vi "Actor Core.vi"(8 "error in":errorcluster, 11 "Stage":refnum<class "Stage.lvclass">) -> (0 "error out":errorcluster, 3 "Actor out":refnum<class "Actor.lvclass">)   [LabVIEW 2018, in "Stage Actor.lvlib" / "Stage.lvclass"]
doc: "This is Actor Core.vi, the main message handling loop for Actors. An actor usually just sits in this loop and processes messages as they arrive. Any error returned by the message Do.vi call will stop the loop, with error code 43 as the canonical signal to stop with no error sent to caller. Descendants may override that in Handle Error.vi."
uses:
  Stage.lvclass
  C:/Program Files (x86)/National Instruments/LabVIEW 2018/vi.lib/MGI/Panel Manager/Panel Actor/Panel Actor/Panel Actor.lvclass
  C:/Program Files (x86)/National Instruments/LabVIEW 2018/vi.lib/ActorFramework/Actor/Actor.lvclass
  <vilib>/ActorFramework/Actor/Actor.lvclass
  Stage.lvclass/Stage.ctl
  <vilib>/ActorFramework/Actor/Actor.lvclass/Actor.ctl
  <vilib>/ActorFramework/Message Enqueuer/Message Enqueuer.lvclass/Message Enqueuer.ctl
  Stage Messages/Set Axis Speed Msg/Set Axis Speed Msg.lvclass/Set Axis Speed Msg.ctl
  Stage Messages/Move to Position Msg/Move to Position Msg.lvclass/Move to Position Msg.ctl
  Stage Messages/Parse Gcode Msg/Parse Coords Msg.lvclass/Parse Coords Msg.ctl
  <vilib>/ActorFramework/Message Enqueuer/Init from Existing Queue.vi
  <vilib>/ActorFramework/Message Enqueuer/Enqueue.vi
  Stage Messages/Stop Stage Msg/Stop Stage Msg.lvclass
  C:/Program Files (x86)/National Instruments/LabVIEW 2018/vi.lib/ActorFramework/Message/Message.lvclass
  Stage Messages/Set Axis Speed Msg/Set Axis Speed Msg.lvclass
  Stage Messages/Home Stage Msg/Home Stage Msg.lvclass
  Stage Messages/Move to Position Msg/Move to Position Msg.lvclass
  Stage Messages/Test VI Msg/Test VI Msg.lvclass
  Stage Messages/Parse Gcode Msg/Parse Coords Msg.lvclass
  <vilib>/ActorFramework/Message Priority Queue/Priority Enqueue.vi
  <vilib>/ActorFramework/Message Enqueuer/Message Enqueuer.lvclass
  <vilib>/MGI/Panel Manager/Panel Actor/Panel Actor/Panel Actor.lvclass
  ADM/Main.lvlib
  <instrlib>/Zaber A Series/Zaber A Series.lvlib
  Stage Messages/Stage Polling Loop Msg/Stage Polling Loop Msg.lvclass
  Stage Messages/Stage Printing Loop Msg/Stage Printing Loop Msg.lvclass
panel:
  in  "Apply Movement":bool
  in  "Travel to Saved":bool
  in  "Save Position":bool
  in  "Move to Specified Position":dbl[](array[numeric])
  out "Saved Position":dbl[](array[numeric])
  in  "Z Speed(mm/s)":dbl(slide)=0.09999999999999998 min=0.0 max=10.0 step=0.01 scale=0.01..10.0
  in  "XY Speed":i16(ring)=10 items=["Fast"=10, "Slow"=1]
  in  "Cancel Button":bool
  in  "Print":bool
  in  "Read Coordinates":path
  in  "-Z":bool
  in  "+Z":bool
  in  "Home Button":bool
  in  "-X":bool
  in  "+X":bool
  in  "-Y":bool
  in  "+Y":bool
  out "Current Position":dbl[](array[numeric])
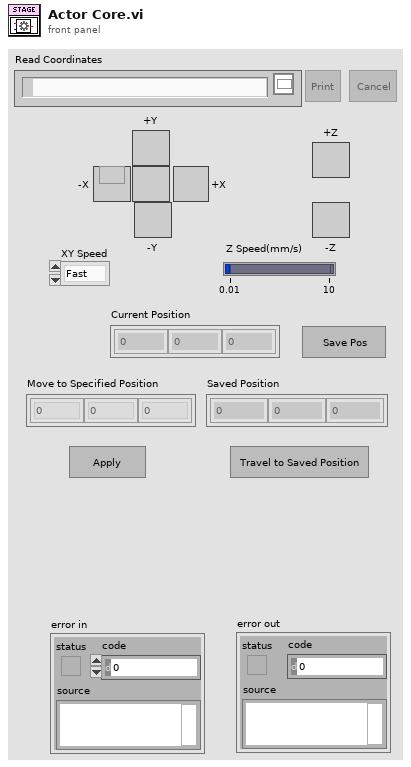
[diagram p1: front panel]
types:
  T1 = cluster{"Print Data":cluster{"XYZ":dbl[][], "Theta Phi":dbl[][], "Current Tool":i16[], "Speed":dbl[], "Feeder State":bool[]}, "Task":string}
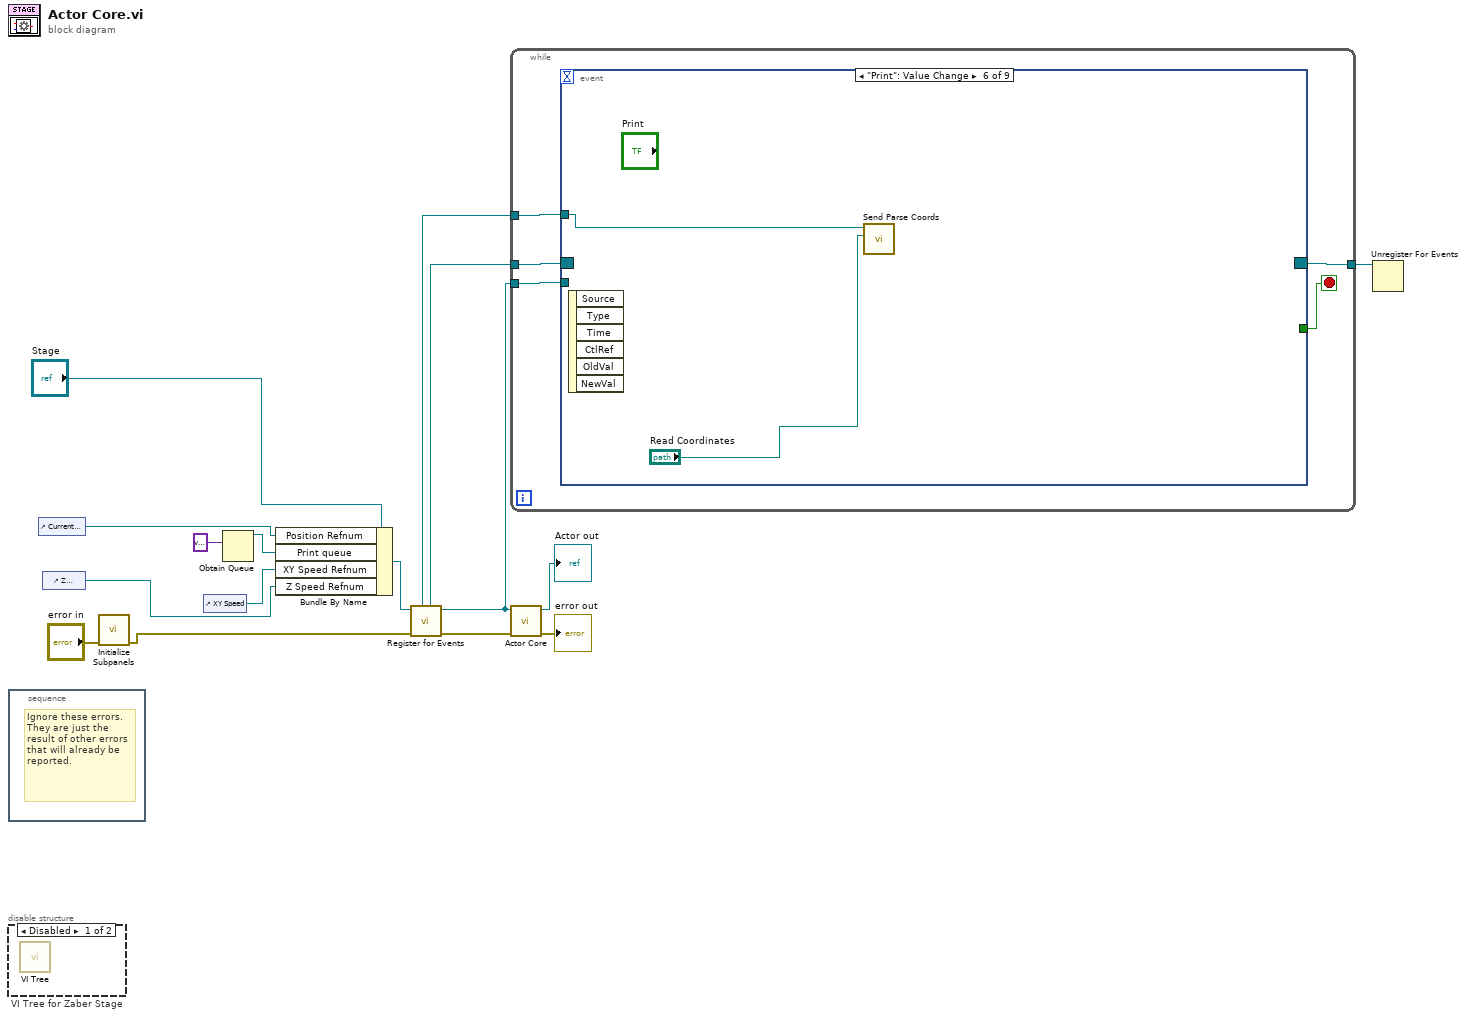
[diagram p0: block diagram]
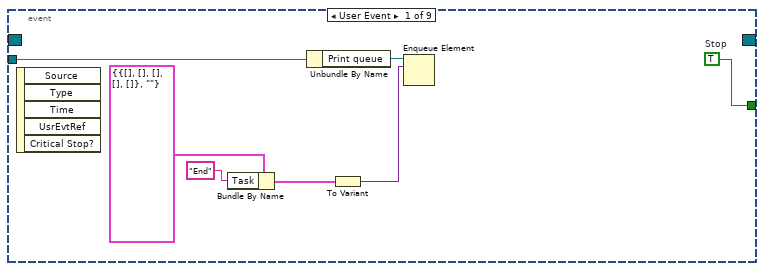
[diagram p2: hidden frame]
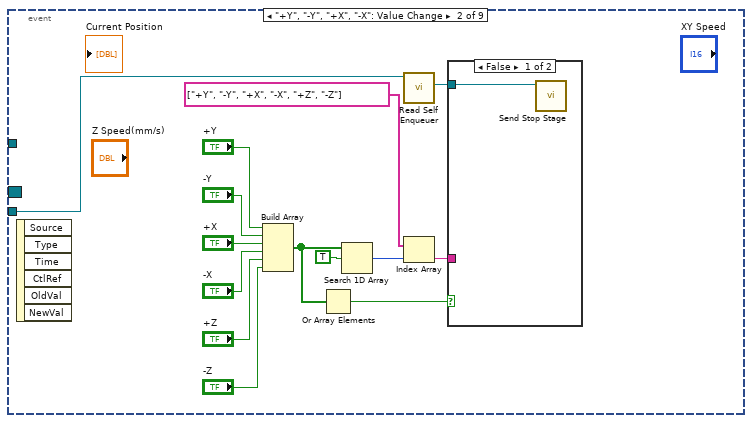
[diagram p3: hidden frame]
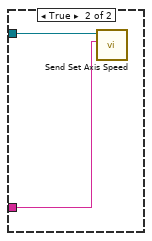
[diagram p4: hidden frame]
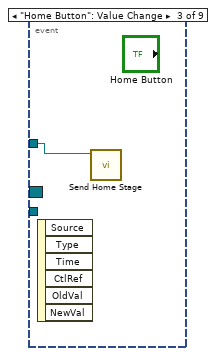
[diagram p5: hidden frame]
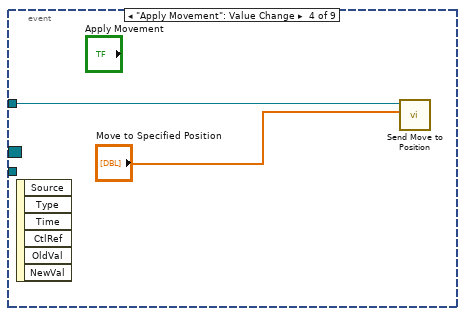
[diagram p6: hidden frame]
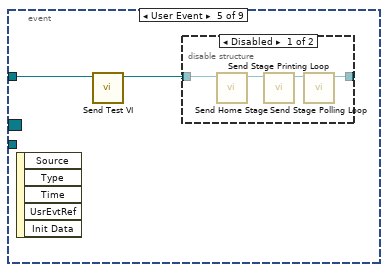
[diagram p7: hidden frame]
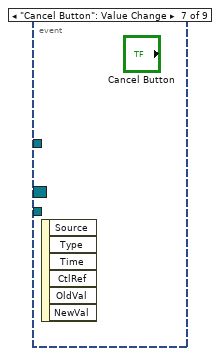
[diagram p9: hidden frame]
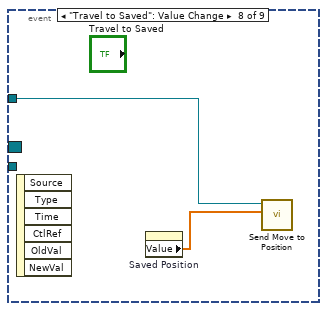
[diagram p10: hidden frame]
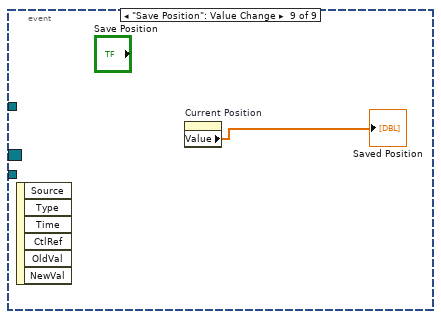
[diagram p11: hidden frame]
diagram:
  n1 = stacked-sequence {
    frame #0 {
      # "Ignore these errors.\nThey are just the result of other errors that will already be reported."
    }
  }
  n2 = disable-structure "VI Tree for Zaber Stage" shown="Disabled" {
    frame Disabled {
      n3 = call <instrlib>:"VI Tree.vi"() -> ()  [unwired: 12 in]
    }
    frame Enabled {
    }
  }
  n4 = control-ref of="Current Position"() -> (w12:refnum<vi>)
  n5 = control-ref of="Z Speed(mm/s)"() -> (w8:refnum<vi>)
  n6 = call "Initialize Subpanels.vi"("error in (no error)"="error in") -> ("error out"=w1:errorcluster)  [unwired: 10 in]
  n7 = control-ref of="XY Speed"() -> (w9:refnum<vi>)
  n8 = Obtain Queue(element data type=variant) -> (queue out=w11:refnum<queue>)  [unwired: 4 in, 2 out]
  n9 = Bundle By Name(cluster="Stage", "Position Refnum"=w12, "Print queue"=w11, "XY Speed Refnum"=w9, "Z Speed Refnum"=w8) -> (w6:refnum<class "Stage.lvclass">)
  n10 = call <vilib>:"Register for Events.vi"("Error In"=w1, "Panel Actor in"=w6) -> ("Error Out"=w5:errorcluster, "Panel Actor out"=w3:refnum<class "Stage.lvclass">, "Pnl Actor"=w4:refnum<event-registration>, "Self Enqueuer"=w2:refnum<class "Message Enqueuer.lvclass">)  [unwired: 6 in]
  n11 = while {
    tunnel: w4 -> [w20]
    tunnel: [w19] -> w14
    tunnel: w3 -> [w18]
    tunnel: w2 -> [w17]
    stop <- w21 stop-if-true
    n12 = event shown="[5] \"Print\": Value Change" {
      selector: w20 -> [_ _ _ _ _ _ _ _ _]
      dyn-events: [_ _ _ _ _ _ _ _ _] -> w19
      timeout: _ -> [_ _ _ _ _ _ _ _ _]
      tunnel: [w28 _ _ _ _ _ _ _ _] -> w21
      tunnel: w18 -> [w27 w30 _ _ _ _ _ _ _]
      tunnel: w17 -> [_ _ w46 w47 w50 w57 _ w59 _]
      event User Event {
        w28 = TRUE  # Stop
        n13 = event-data() -> ()  [unwired: 1 in, 5 out]
        n14 = Bundle By Name(cluster=T1 {"Print Data"={"XYZ"=[], "Theta Phi"=[], "Current Tool"=[], "Speed"=[], "Feeder State"=[]}, "Task"=""} ("Print Message"), "Task"="End") -> (w23:T1)
        n15 = Unbundle By Name(w27) -> ("Print queue"=w26:refnum<queue>)
        n16 = To Variant(anything=w23) -> (Variant=w22:variant)
        n17 = Enqueue Element(queue=w26, element=w22) -> ()  [unwired: 2 in, 3 out]
      }
      event "+Y", "-Y", "+X", "-X": Value Change {
        n18 = event-data() -> ()  [unwired: 1 in, 6 out]
        n19 = Build Array("+Y", "-Y", "+X", "-X", "+Z", "-Z") -> (w37:bool[])
        n20 = Or Array Elements(Boolean array=w37) -> (logical OR=w38:bool)
        n21 = Search 1D Array(1D array=w37, element=TRUE) -> (index of element=w35:i32)  [unwired: 1 in]
        n22 = call <vilib>:"Read Self Enqueuer.vi"("Actor"=w30) -> ("Self Enqueuer"=w29:refnum<class "Message Enqueuer.lvclass">)  [unwired: 10 in]
        n23 = Index Array(array=string[] ["+Y", "-Y", "+X", "-X", "+Z", "-Z"], index=w35) -> (element=w33:string)
        n24 = case shown="False" w38 {
          tunnel: w33 -> [_ w45]
          tunnel: w29 -> [w43 w44]
          frame False {
            n25 = call "Send Stop Stage.vi"("Message Enqueuer"=w43) -> ()  [unwired: 9 in, 2 out]
          }
          frame True {
            n26 = call "Send Set Axis Speed.vi"("Axis"=w45, "Message Enqueuer"=w44) -> ()  [unwired: 8 in, 2 out]
          }
        }
      }
      event "Home Button": Value Change {
        n27 = event-data() -> ()  [unwired: 1 in, 6 out]
        n28 = call "Send Home Stage.vi"("Message Enqueuer"=w46) -> ()  [unwired: 9 in, 2 out]
      }
      event "Apply Movement": Value Change {
        n29 = event-data() -> ()  [unwired: 1 in, 6 out]
        n30 = call "Send Move to Position.vi"("Position"="Move to Specified Position", "Message Enqueuer"=w47) -> ()  [unwired: 8 in, 2 out]
      }
      event User Event {
        n31 = event-data() -> ()  [unwired: 1 in, 5 out]
        n32 = call "Send Test VI.vi"("Message Enqueuer"=w50) -> ("Message Enqueuer out"=w49:refnum<class "Message Enqueuer.lvclass">)  [unwired: 9 in, 1 out]
        n33 = disable-structure shown="Disabled" {
          disable-tunnel: w49 -> [w52 w55]
          disable-tunnel: [w53 w55] -> _
          frame Disabled {
            n34 = call "Send Home Stage.vi"("Message Enqueuer"=w52) -> ("Message Enqueuer out"=w51:refnum<class "Message Enqueuer.lvclass">)  [unwired: 9 in, 1 out]
            n35 = call "Send Stage Printing Loop.vi"("Message Enqueuer"=w51) -> ("Message Enqueuer out"=w54:refnum<class "Message Enqueuer.lvclass">)  [unwired: 9 in, 1 out]
            n36 = call "Send Stage Polling Loop.vi"("Message Enqueuer"=w54) -> ("Message Enqueuer out"=w53:refnum<class "Message Enqueuer.lvclass">)  [unwired: 9 in, 1 out]
          }
          frame Enabled {
          }
        }
      }
      event "Print": Value Change {
        n37 = event-data() -> ()  [unwired: 1 in, 6 out]
        n38 = call "Send Parse Coords.vi"("Read Coordinates"="Read Coordinates", "Message Enqueuer"=w57) -> ()  [unwired: 8 in, 2 out]
      }
      event "Cancel Button": Value Change {
        n39 = event-data() -> ()  [unwired: 1 in, 6 out]
      }
      event "Travel to Saved": Value Change {
        n40 = event-data() -> ()  [unwired: 1 in, 6 out]
        n41 = property on="Saved Position" class="Arr (strict)"() -> ("Value"=w58:dbl[])  [unwired: 2 in, 2 out]
        n42 = call "Send Move to Position.vi"("Position"=w58, "Message Enqueuer"=w59) -> ()  [unwired: 8 in, 2 out]
      }
      event "Save Position": Value Change {
        n43 = event-data() -> ()  [unwired: 1 in, 6 out]
        n44 = property on="Current Position" class="Arr (strict)"() -> ("Value"=→"Saved Position":dbl[])  [unwired: 2 in, 2 out]
      }
    }
  }
  n45 = call-parent "Actor Core.vi"("error in"=w5, "Panel Actor in"=w3) -> ("error out"=→"error out":errorcluster, "Actor out"=→"Actor out":refnum<class "Actor.lvclass">)  [unwired: 8 in]
  n46 = Unregister For Events(event registration refnum=w14) -> ()  [unwired: 1 in, 1 out]
